vi "DoCreate.vi"(8 "ErrorIn":errorcluster, 11 "ReferenceIn":refnum<class "YAFTAF.lvclass">) -> (0 "ErrorOut":errorcluster, 3 "ReferenceOut":refnum<class "YAFTAF.lvclass">)   [LabVIEW 2021, in "YAFTAF.lvclass"]
uses:
  YAFTAF.lvclass
  YAFTAF.lvclass/YAFTAF.ctl
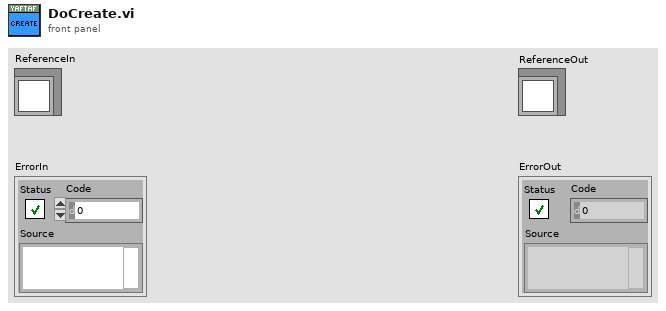
[diagram p1: front panel]
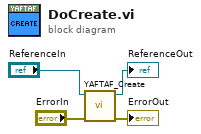
[diagram p0: block diagram]
diagram:
  n1 = call-dynamic "YAFTAF_Create.vi"("Error In"="ErrorIn", "object in"="ReferenceIn") -> ("Error Out"=→"ErrorOut":errorcluster, "object out"=→"ReferenceOut":refnum<class "YAFTAF.lvclass">)  [unwired: 8 in]
